vi "Unflatten Value.vi"(0 "Float In":refnum<class "Float.lvclass">, 7 "Value":string, 11 "Error In":errorcluster) -> (4 "Float Out":refnum<class "Float.lvclass">, 15 "Error Out":errorcluster)   [LabVIEW 2016, in "Float.lvclass"]
uses:
  Float.lvclass
  Float.lvclass/Float.ctl
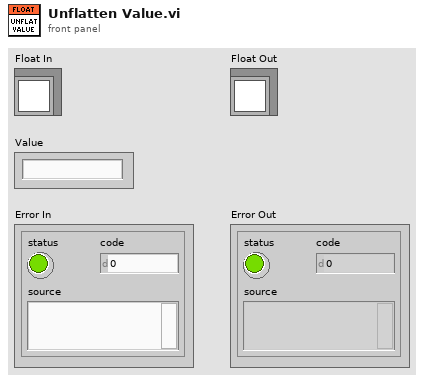
[diagram p1: front panel]
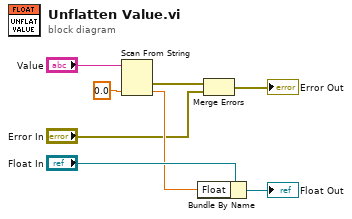
[diagram p0: block diagram]
diagram:
  n1 = Scan From String(input string="Value", default 1=0.0 ("default value 1")) -> (error out=w3:errorcluster, output 1=w4:dbl)  [unwired: 3 in, 2 out]
  n2 = Bundle By Name(cluster="Float In", "Float"=w4) -> (→"Float Out":refnum<class "Float.lvclass">)
  n3 = Merge Errors(w3, "Error In") -> (→"Error Out":errorcluster)
